vi "OAT Compensate Even Angle Signal (Vector Ref, 1 Channel).vi"(0 "even-angle signal":cluster{"r0":dbl, "dr":dbl, "Y":dbl[]}={"r0"=0.0, "dr"=1.0, "Y"=[]} {"r0" format="%.2p"; "dr" format="%.2p"; "Y" format="%.2f"}, 1 "orders to compensate":dbl[](array[numeric]) format="%.2f", 2 "reset? (F)":bool, 5 "vector references":cdb[](array[numeric]) format="%.2f", 7 "even-angle position info":T1, 9 "speed profile":T2 {"speed [RPM]" format="%.2f"; "time [s]" format="%.2f"}, 11 "error in (no error)":errorcluster) -> (4 "compensated even-angle signal":cluster{"r0":dbl, "dr":dbl, "Y":dbl[]}={"r0"=0.0, "dr"=1.0, "Y"=[]} {"r0" format="%.2p"; "dr" format="%.2p"; "Y" format="%.2f"}, 6 "actual vector references":cdb[](array[numeric]) format="%.2f", 8 "even-angle position info out":T1, 15 "error out":errorcluster)   [LabVIEW 2017, in "SoundVib_RefDataProcess.lvlib"]
doc: "Compensates an even-angle signal. You can use the <B>compensated even-angle signal</B> output to display unfiltered orbit and timebase plots with the runout pattern removed. Wire data to the <B>even-angle signal</B> input to determine the polymorphic instance to use or manually select the instance."
uses:
  <vilib>/addons/Sound and Vibration/Order Analysis/Referece Data Processing/SoundVib_RefDataProcess.lvlib
  <vilib>/addons/Sound and Vibration/Order Analysis/Misc/OAT Position Info.ctl
  <vilib>/addons/Sound and Vibration/Order Analysis/Tach Process/SubVIs/speed profile.ctl
  <vilib>/addons/Sound and Vibration/Order Analysis/Resample Order Tracking/SoundVib_Resampling.lvlib
  <vilib>/addons/Sound and Vibration/Order Analysis/Tach Process/SoundVib_TachProcess.lvlib
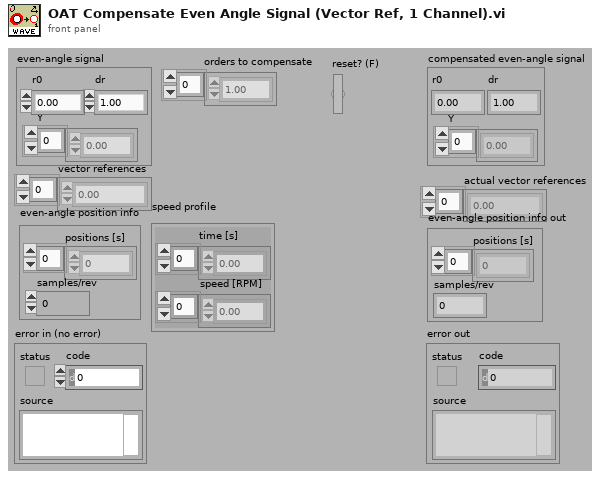
[diagram p1: front panel]
types:
  T1 = typedef "OAT Position Info.ctl" = cluster{"positions [s]":dbl[], "samples/rev":dbl}
  T2 = typedef "SoundVib_TachProcess.lvlib/speed profile.ctl" = cluster{"time [s]":dbl[], "speed [RPM]":dbl[]}
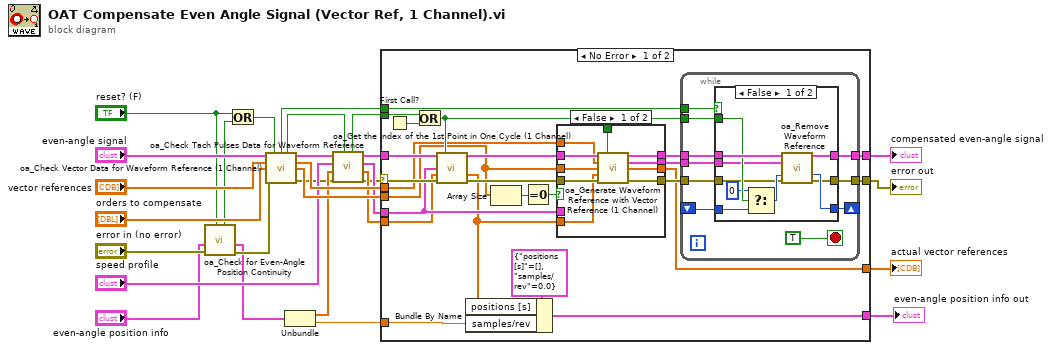
[diagram p0: block diagram]
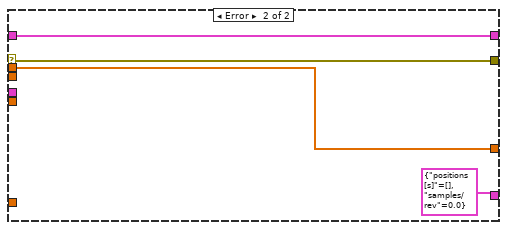
[diagram p4: hidden frame]
diagram:
  n1 = call <vilib>:"oa_Check for Even-Angle Position Continuity.vi"("reset in"="reset? (F)", "error in (no error)"="error in (no error)", "even-angle position info"="even-angle position info") -> ("error out"=w6:errorcluster, "even-angle position info dup"=w4:T1, "position not continuous"=w2:bool)  [unwired: 6 in]
  n2 = Or(x="reset? (F)", y=w2) -> (x .or. y?=w1:bool)
  n3 = call <vilib>:"oa_Check Vector Data for Waveform Reference (1 Channel).vi"("resampled signal"="even-angle signal", "reset? (True)"=w1, "slow roll vectors"="vector references", "orders to compensate"="orders to compensate", "error out in"=w6) -> ("empty signal?"=w10:bool, "parameter changed"=w12:bool, "resampled signal dup"=w20:cluster{"r0":dbl, "dr":dbl, "Y":dbl[]}, "slow roll vectors dup"=w25:cdb[], "orders to compensate dup"=w24:dbl[], "error out"=w14:errorcluster)  [unwired: 5 in]
  n4 = Unbundle(w4) -> ("positions [s]"=w16:dbl[], "samples/rev"=w9:dbl)
  n5 = call <vilib>:"oa_Check Tach Pulses Data for Waveform Reference.vi"("reset? (True)"=w12, "error in (no error)"=w14, "interpolated pulse positions"=w16, "speed profile"="speed profile", "resampled signal"=w20) -> ("error out"=w13:errorcluster, "interpolated pulse positions out"=w15:dbl[], "speed profile out"=w17:T2, "resampled signal out"=w19:cluster{"r0":dbl, "dr":dbl, "Y":dbl[]}, "reset"=w11:bool)  [unwired: 2 in]
  n6 = case shown="No Error" w13 {
    selector: w13 -> [w51 w90]
    tunnel: w25 -> [w36 w91]
    tunnel: w24 -> [w39 _]
    tunnel: w19 -> [w52 w92]
    tunnel: [w50 w92] -> w23
    tunnel: [w35 w91] -> w22
    tunnel: [w49 w90] -> w21
    tunnel: w17 -> [w45 _]
    tunnel: w15 -> [w33 _]
    tunnel: w11 -> [w40 _]
    tunnel: w10 -> [w34 _]
    tunnel: w9 -> [w31 _]
    tunnel: [w29 T1 {"positions [s]"=[], "samples/rev"=0.0} ("even angle position info")] -> w8
    frame No Error {
      n7 = First Call?() -> (First Call?: T/F=w42:bool)
      n8 = Or(x=w40, y=w42) -> (x .or. y?=w41:bool)
      n9 = call <vilib>:"oa_Get the Index of the 1st Point in One Cycle (1 Channel).vi"("resampled signal"=w52, "reset? (True)"=w41, "speed profile"=w45, "interpolated pulse positions"=w33, "error in (no error)"=w51) -> ("resampled signal out"=w48:cluster{"r0":dbl, "dr":dbl, "Y":dbl[]}, "interpolated pulse positions out"=w30:dbl[], "error out"=w47:errorcluster)  [unwired: 8 in]
      n10 = Bundle By Name(cluster=T1 {"positions [s]"=[], "samples/rev"=0.0} ("even angle position info"), "positions [s]"=w30, "samples/rev"=w31) -> (w29:T1)
      n11 = Array Size(array=w39) -> (size(s)=w43:i32)
      n12 = Equal To 0?(x=w43) -> (x = 0?=w44:bool)
      n13 = case shown="False" w44 {
        tunnel: w48 -> [w62 w63]
        tunnel: w47 -> [w61 w64]
        tunnel: [w60 w63] -> w37
        tunnel: [w59 w64] -> w46
        tunnel: [w58 _] -> w38
        tunnel: w36 -> [w57 w65]
        tunnel: w39 -> [w56 _]
        tunnel: w45 -> [_ _]
        tunnel: w30 -> [w54 _]
        tunnel: w41 -> [w55 _]
        tunnel: [w53 w65] -> w35
        frame False {
          n14 = call <vilib>:"oa_Generate Waveform Reference with Vector Reference (1 Channel).vi"("resampled signal"=w62, "reset? (True)"=w55, "slow roll vectors"=w57, "orders to compensate"=w56, "interpolated pulse positions"=w54, "error out in"=w61) -> ("resampled signal out"=w60:cluster{"r0":dbl, "dr":dbl, "Y":dbl[]}, "baseline in"=w58:cluster{"r0":dbl, "dr":dbl, "Y":dbl[]}, "slow roll vectors out"=w53:cdb[], "error out"=w59:errorcluster)  [unwired: 6 in]
        }
        frame True {
        }
      }
      n15 = while {
        shift-right: [w72] -> _
        shift-left: _ -> [w71]
        tunnel: w41 -> [w73]
        tunnel: w46 -> [w70]
        tunnel: [w69] -> w49
        tunnel: w38 -> [w67]
        tunnel: w34 -> [w66]
        tunnel: w37 -> [w75]
        tunnel: [w68] -> w50
        stop <- TRUE stop-if-true
        n16 = case shown="False" w66 {
          tunnel: w75 -> [w85 w88]
          tunnel: w73 -> [w84 _]
          tunnel: [w83 w86] -> w72
          tunnel: w71 -> [w82 w86]
          tunnel: w70 -> [w79 w87]
          tunnel: [w78 w87] -> w69
          tunnel: [w77 w88] -> w68
          tunnel: w67 -> [w76 _]
          frame False {
            n17 = Select(t=0, s=w84, f=w82) -> (s? t:f=w80:i32)
            n18 = call <vilib>:"oa_Remove Waveform Reference.vi"("resampled signal"=w85, "baseline in"=w76, "last index"=w80, "error out in"=w79) -> ("compensated signal"=w77:cluster{"r0":dbl, "dr":dbl, "Y":dbl[]}, "last index out"=w83:i32, "error out"=w78:errorcluster)  [unwired: 9 in]
          }
          frame True {
          }
        }
      }
    }
    frame Error {
    }
  }
  "compensated even-angle signal" <- w23
  "error out" <- w21
  "actual vector references" <- w22
  "even-angle position info out" <- w8
